vi "axis x.vi"() -> ()   [LabVIEW 2015]
panel:
  in  "Freq":dbl=1.0 min=0.001 format="%#_6p"
  out "error out":errorcluster
  in  "error in (no error)":errorcluster
  out "VISA resource name 2":refnum<visa-resource-name>
  in  "VISA resource name":refnum<visa-resource-name>
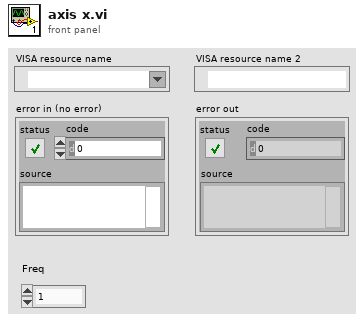
[diagram p1: front panel]
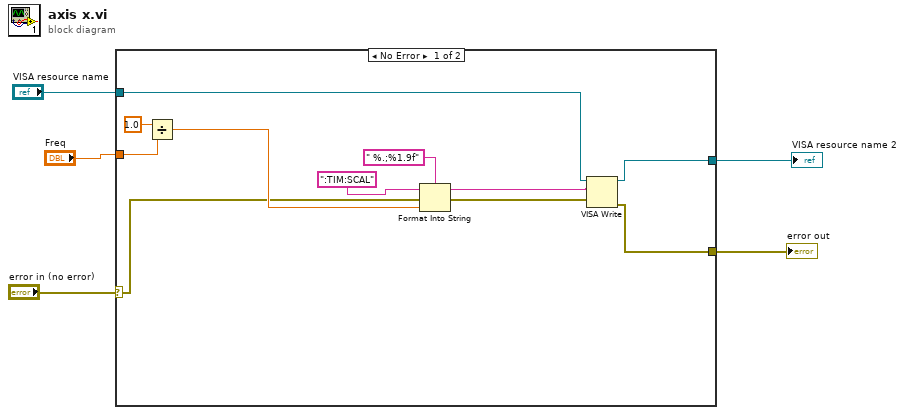
[diagram p0: block diagram]
diagram:
  n1 = case shown="No Error" "error in (no error)" {
    selector: "error in (no error)" -> [w8 w18]
    tunnel: "VISA resource name" -> [w10 w17]
    tunnel: "Freq" -> [w16 _]
    tunnel: [w7 _] -> w2
    tunnel: [w6 _] -> w1
    frame No Error {
      n2 = Divide(x=1.0, y=w16) -> (x/y=w9:dbl)
      n3 = Format Into String(format string=" %.;%1.9f", initial string=":TIM:SCAL", error in=w8, w9) -> (resulting string=w14:string, error out=w13:errorcluster)
      n4 = VISA Write(VISA resource name=w10, write buffer=w14, error in (no error)=w13) -> (VISA resource name out=w7:refnum<visa-resource-name>, error out=w6:errorcluster)  [unwired: 1 out]
    }
    frame Error {
    }
  }
  "VISA resource name 2" <- w2
  "error out" <- w1
